vi "GetPageSelectorReference.vi"(8 "error in":errorcluster, 11 "PageSelector in":refnum<class "PageSelector.lvclass">) -> (0 "error out":errorcluster, 1 "page selector reference":refnum<vi>, 3 "PageSelector out":refnum<class "PageSelector.lvclass">)   [LabVIEW 2014, in "Raspberry Pi Compatible Compiler for LabVIEW.lvlib" / "PageSelector.lvclass"]
uses:
  PageSelector.lvclass
  Generic/Generic.lvclass
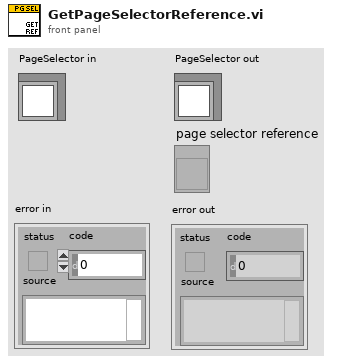
[diagram p1: front panel]
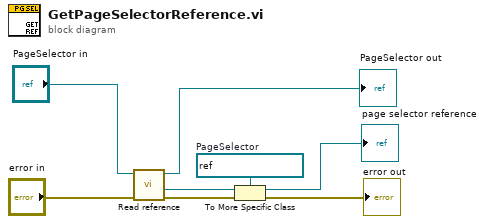
[diagram p0: block diagram]
diagram:
  w6 = refnum<vi> refnum  # PageSelector
  n1 = call "Read reference.vi"("error in"="error in", "GObject in"="PageSelector in") -> ("error out"=w7:errorcluster, "reference"=w8:refnum<vi>, "GObject out"=→"PageSelector out":refnum<class "PageSelector.lvclass">)  [unwired: 5 in]
  n2 = To More Specific Class(target class=w6, reference=w8, error in=w7) -> (specific class reference=→"page selector reference":refnum<vi>, error out=→"error out":errorcluster)
